vi "Rosie-Load-Keywords.vi"() -> (2 "Diodes Keywords Array":T1[](array[typedef]))   [LabVIEW 2020]
uses:
  Common/DolphinDAQ-SCPI-Driver/DDAQ-Keyword.ctl
panel:
  out "Path to Keywords CSV":path
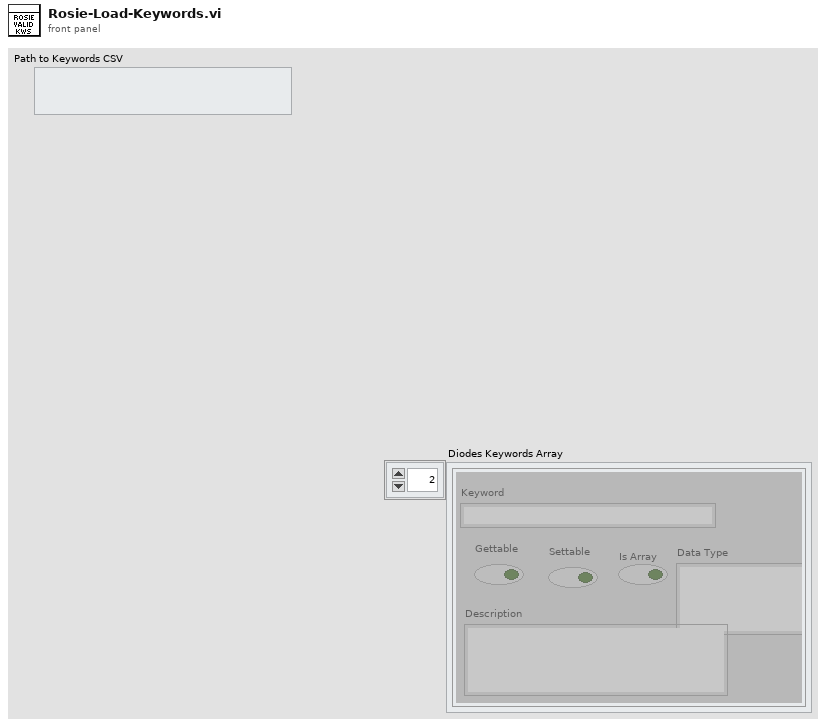
[diagram p1: front panel]
types:
  T1 = typedef "DDAQ-Keyword.ctl" = cluster{"Keyword":string, "Gettable":bool, "Settable":bool, "Is Array":bool, "Data Type":string, "Description":string}
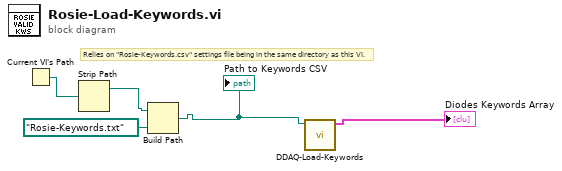
[diagram p0: block diagram]
diagram:
  # "Relies on \"Rosie-Keywords.csv\" settings file being in the same directory as this VI."
  n1 = Current VI's Path() -> (path=w4:path)
  n2 = Strip Path(path=w4) -> (stripped path=w3:path)  [unwired: 1 out]
  n3 = Build Path(base path=w3, name or relative path=path "Rosie-Keywords.txt") -> (appended path=w2:path)
  "Path to Keywords CSV" <- w2
  n4 = call "DDAQ-Load-Keywords.vi"("Path to Keywords CSV"=w2) -> ("Diodes Keywords Array"=→"Diodes Keywords Array":T1[])  [unwired: 10 in]
